vi "OverrideVI.vi"(8 "error in (no error)":errorcluster, 10 "Name":string, 11 "CreateClass In":refnum<class "CreateClass.lvclass">) -> (0 "error out":errorcluster, 3 "CreateClass Out":refnum<class "CreateClass.lvclass">)   [LabVIEW 2020, in "Mermaid.lvlib" / "CreateClass.lvclass"]
uses:
  CreateClass.lvclass
  CreateClass.lvclass/CreateClass.ctl
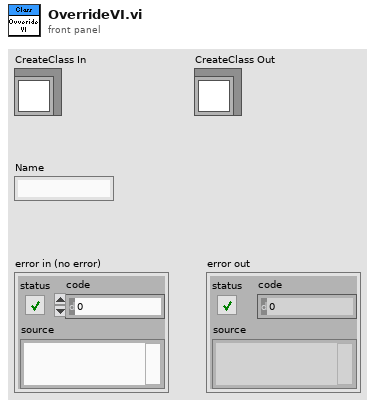
[diagram p1: front panel]
types:
  T1 = enum32{"invalid VI type", "Standard VI", "Control VI", "Global VI", "Polymorphic VI", "Configuration VI", "SubSystem", "Facade VI", "Method VI", "Statechart Diagram VI"}
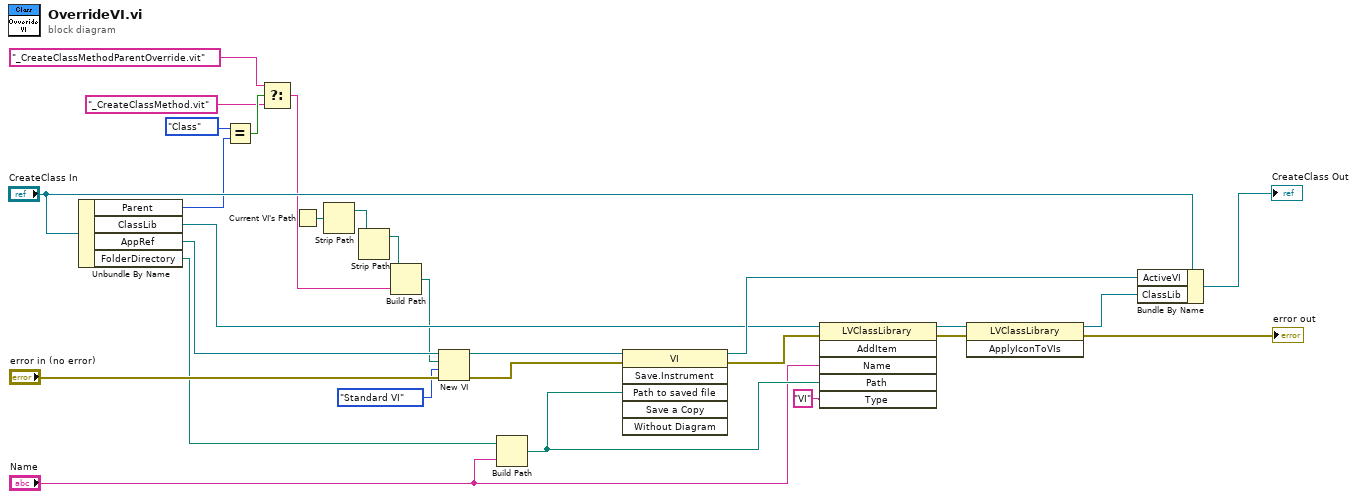
[diagram p0: block diagram]
diagram:
  n1 = Unbundle By Name("CreateClass In") -> ("Parent"=w10:enum16{"None", "Interface", "Class"}, "ClassLib"=w25:refnum<vi>, "AppRef"=w24:refnum<vi>, "FolderDirectory"=w14:path)
  n2 = Equal?(x=enum16{"None", "Interface", "Class"}."Class", y=w10) -> (x = y?=w11:bool)
  n3 = Select(t="_CreateClassMethodParentOverride.vit" ("Name"), s=w11, f="_CreateClassMethod.vit" ("Name")) -> (s? t:f=w6:string)
  n4 = Current VI's Path() -> (path=w5:path)
  n5 = Strip Path(path=w5) -> (stripped path=w3:path)  [unwired: 1 out]
  n6 = Strip Path(path=w3) -> (stripped path=w2:path)  [unwired: 1 out]
  n7 = Build Path(base path=w2, name or relative path=w6) -> (appended path=w4:path)
  n8 = New VI(8:"error in (no error)", 9:T1."Standard VI" ("vi type (standard vi)"), 10:w4, 11:w24) -> (0:w16:errorcluster, 3:w15:refnum<vi>)  [unwired: 3 in]
  n9 = Build Path(base path=w14, name or relative path="Name") -> (appended path=w18:path)
  n10 = invoke class="VI" method="Save.Instrument"(reference=w15, error in=w16, "Path to saved file"=w18) -> (reference out=w26:refnum<vi>, error out=w17:errorcluster)  [unwired: 3 in, 4 out]
  n11 = invoke class="LVClassLibrary" method="AddItem"(reference=w25, error in=w17, "Name"="Name", "Path"=w18, "Type"="VI") -> (reference out=w21:refnum<vi>, error out=w22:errorcluster)  [unwired: 1 in, 4 out]
  n12 = invoke class="LVClassLibrary" method="ApplyIconToVIs"(reference=w21, error in=w22) -> (reference out=w28:refnum<vi>, error out=→"error out":errorcluster)  [unwired: 1 in, 1 out]
  n13 = Bundle By Name(cluster="CreateClass In", "ActiveVI"=w26, "ClassLib"=w28) -> (→"CreateClass Out":refnum<class "CreateClass.lvclass">)
